vi "Facade.vi"(0 "Data In":T5, 2 "Display State In":T3, 3 "Container State":T4) -> (6 "Data Out":T5, 7 "Display State Out":T3, 8 "Action":T2)   [LabVIEW 2020, in "Termination XCtrl.xctl"]
uses:
  Termination XCtrl.xctl
  <vilib>/_xctls/Action.ctl
  <vilib>/_xctls/XControlSupport.lvlib
  Classes/Termination/Termination.lvclass
  <vilib>/_xctls/Container State.ctl
  Data.vi
  State.vi
panel:
  in  "Color Box":u32(colorbox)
  in  "Result":string
  in  "Tab":enum32{"End", "Finish", "TTL"}(tab)
  in  "Tmin":dbl caption="but wait at least (ms)" min=0.0 step=1.0
  in  "End on rep?":bool caption="end on rep boundary"
  in  "Tttl":string caption="min interval (ms)"
  in  "Nttl":i32 caption="max triggers" min=0 step=1
  in  "TermAction":T1(ring) caption="When true"
  in  "Latency":dbl caption="Response latency (ms)" min=0.0 step=1.0
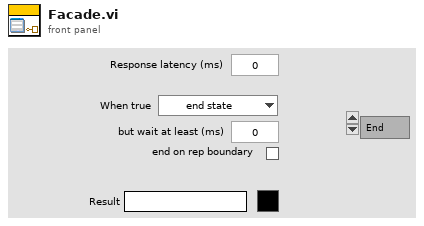
[diagram p1: front panel]
types:
  T1 = enum16{"end state", "let state finish", "TTL only"}
  T2 = typedef "XControlSupport.lvlib/Action.ctl" = cluster{"Data Changed?":bool, "State Changed?":bool, "Action Name":string}
  T3 = typedef "Termination XCtrl.xctl/State.vi" = cluster{"Numeric":dbl}
  T4 = typedef "XControlSupport.lvlib/Container State.ctl" = cluster{"Indicator?":bool, "Run Mode?":bool, " Refnum":refnum<vi>}
  T5 = typedef "Termination XCtrl.xctl/Data.vi" = refnum<class "Termination.lvclass">
  T6 = typedef "Tosca-Termination Condition Action.ctl" = enum16{"End state", "Complete state", "TTL only"}
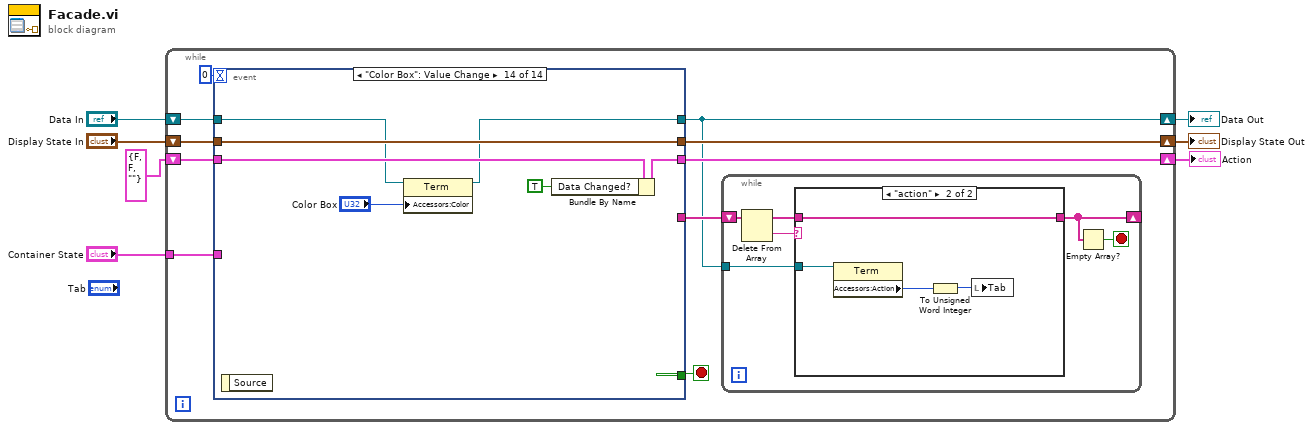
[diagram p0: block diagram]
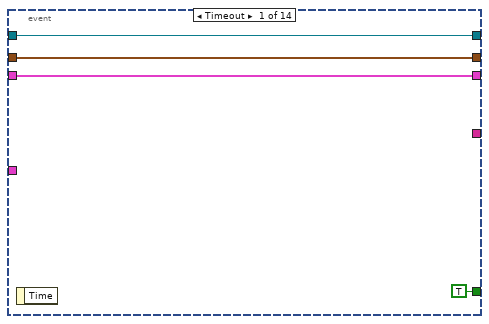
[diagram p3: hidden frame]
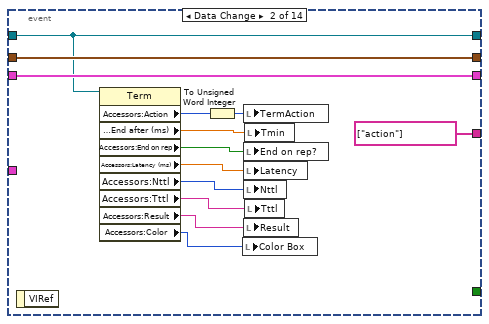
[diagram p4: hidden frame]
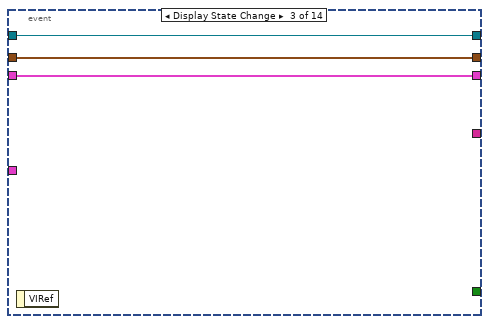
[diagram p5: hidden frame]
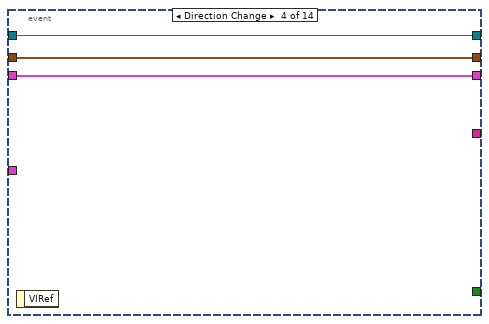
[diagram p6: hidden frame]
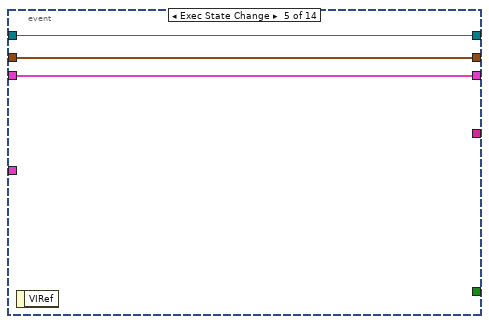
[diagram p7: hidden frame]
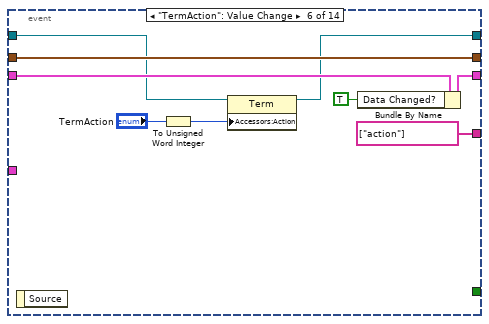
[diagram p8: hidden frame]
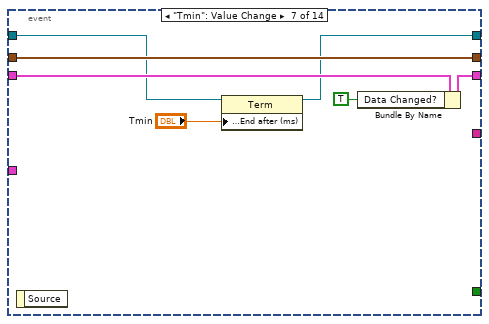
[diagram p9: hidden frame]
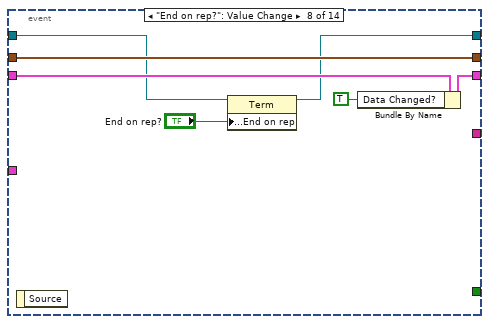
[diagram p10: hidden frame]
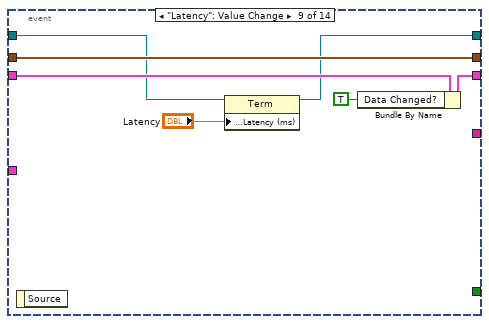
[diagram p11: hidden frame]
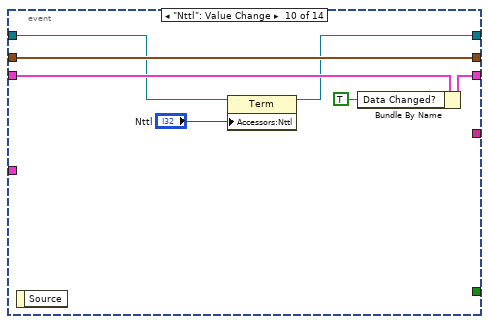
[diagram p12: hidden frame]
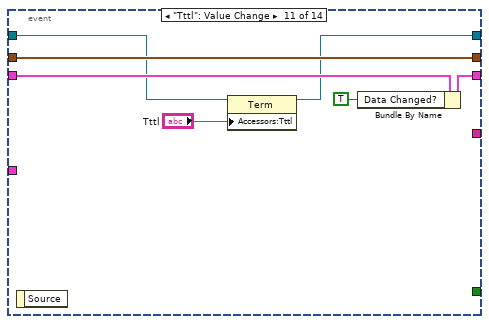
[diagram p13: hidden frame]
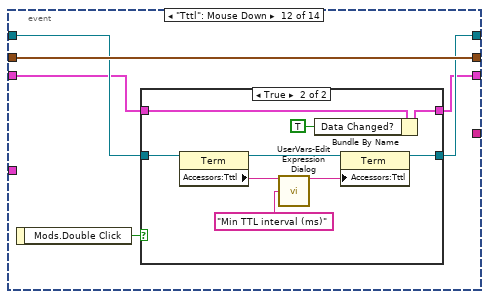
[diagram p14: hidden frame]
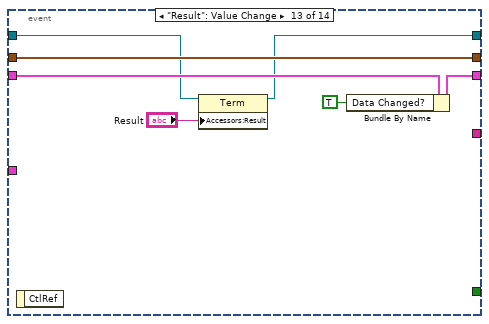
[diagram p16: hidden frame]
diagram:
  n1 = while {
    shift-right: [w16] -> w4
    shift-left: "Display State In" -> [w17]
    tunnel: "Container State" -> [w13]
    shift-right: [w8] -> w7
    shift-left: "Data In" -> [w12]
    shift-right: [w10] -> w2
    shift-left: T2 {"Data Changed?"=FALSE, "State Changed?"=FALSE, "Action Name"=""} ("Action") -> [w11]
    stop <- w15 stop-if-true
    n2 = event shown="[13] \"Color Box\": Value Change" {
      selector: _ -> [_ _ _ _ _ _ _ _ _ _ _ _ _ _]
      dyn-events: _ -> [_ _ _ _ _ _ _ _ _ _ _ _ _ _]
      timeout: 0 -> [_ _ _ _ _ _ _ _ _ _ _ _ _ _]
      tunnel: w17 -> [w31 w45 w48 w51 w54 w63 w70 w77 w84 w91 w98 w104 w122 w129]
      tunnel: [w31 w45 w48 w51 w54 w63 w70 w77 w84 w91 w98 w104 w122 w129] -> w16
      tunnel: [TRUE _ _ _ _ _ _ _ _ _ _ _ _ _] -> w15
      tunnel: w13 -> [_ _ _ _ _ _ _ _ _ _ _ _ _ _]
      tunnel: w12 -> [w29 w35 w47 w50 w53 w58 w66 w73 w80 w87 w94 w102 w119 w127]
      tunnel: [w29 w35 w47 w50 w53 w57 w65 w72 w79 w86 w93 w101 w118 w126] -> w8
      tunnel: [w30 w44 w46 w49 w52 w60 w68 w75 w82 w89 w96 w99 w117 w125] -> w10
      tunnel: w11 -> [w30 w44 w46 w49 w52 w62 w69 w76 w83 w90 w97 w100 w121 w128]
      tunnel: [_ string[] ["action"] _ _ _ string[] ["action"] _ _ _ _ _ _ _ _] -> w9
      event Timeout {
        n3 = event-data() -> ()  [unwired: 1 in, 1 out]
      }
      event Data Change {
        n4 = event-data() -> ()  [unwired: 1 in, 1 out]
        n5 = property class="Term"(reference=w35) -> ("Accessors:Action"=w42:T6, "Accessors:End after (ms)"=w39:dbl, "Accessors:End on rep"=w38:bool, "Accessors:Latency (ms)"=w37:dbl, "Accessors:Nttl"=w36:i32, "Accessors:Tttl"=w40:string, "Accessors:Result"=w34:string, "Accessors:Color"=w33:u32)  [unwired: 1 in, 2 out]
        n6 = To Unsigned Word Integer(number=w42) -> (unsigned 16bit integer=w41:u16)
        n7 = local write "Color Box"(w33) -> ()
        n8 = local write "TermAction"(w41) -> ()
        n9 = local write "End on rep?"(w38) -> ()
        n10 = local write "Latency"(w37) -> ()
        n11 = local write "Nttl"(w36) -> ()
        n12 = local write "Result"(w34) -> ()
        n13 = local write "Tmin"(w39) -> ()
        n14 = local write "Tttl"(w40) -> ()
      }
      event Display State Change {
        n15 = event-data() -> ()  [unwired: 1 in, 1 out]
      }
      event Direction Change {
        n16 = event-data() -> ()  [unwired: 1 in, 1 out]
      }
      event Exec State Change {
        n17 = event-data() -> ()  [unwired: 1 in, 1 out]
      }
      event "TermAction": Value Change {
        n18 = event-data() -> ()  [unwired: 1 in, 1 out]
        n19 = To Unsigned Word Integer(number="TermAction") -> (unsigned 16bit integer=w55:u16)
        n20 = property class="Term"(reference=w58, "Accessors:Action"=w55) -> (reference out=w57:T5)  [unwired: 1 in, 1 out]
        n21 = Bundle By Name(cluster=w62, "Data Changed?"=TRUE) -> (w60:T2)
      }
      event "Tmin": Value Change {
        n22 = event-data() -> ()  [unwired: 1 in, 1 out]
        n23 = property class="Term"(reference=w66, "Accessors:End after (ms)"="Tmin") -> (reference out=w65:T5)  [unwired: 1 in, 1 out]
        n24 = Bundle By Name(cluster=w69, "Data Changed?"=TRUE) -> (w68:T2)
      }
      event "End on rep?": Value Change {
        n25 = event-data() -> ()  [unwired: 1 in, 1 out]
        n26 = property class="Term"(reference=w73, "Accessors:End on rep"="End on rep?") -> (reference out=w72:T5)  [unwired: 1 in, 1 out]
        n27 = Bundle By Name(cluster=w76, "Data Changed?"=TRUE) -> (w75:T2)
      }
      event "Latency": Value Change {
        n28 = event-data() -> ()  [unwired: 1 in, 1 out]
        n29 = property class="Term"(reference=w80, "Accessors:Latency (ms)"="Latency") -> (reference out=w79:T5)  [unwired: 1 in, 1 out]
        n30 = Bundle By Name(cluster=w83, "Data Changed?"=TRUE) -> (w82:T2)
      }
      event "Nttl": Value Change {
        n31 = event-data() -> ()  [unwired: 1 in, 1 out]
        n32 = property class="Term"(reference=w87, "Accessors:Nttl"="Nttl") -> (reference out=w86:T5)  [unwired: 1 in, 1 out]
        n33 = Bundle By Name(cluster=w90, "Data Changed?"=TRUE) -> (w89:T2)
      }
      event "Tttl": Value Change {
        n34 = event-data() -> ()  [unwired: 1 in, 1 out]
        n35 = property class="Term"(reference=w94, "Accessors:Tttl"="Tttl") -> (reference out=w93:T5)  [unwired: 1 in, 1 out]
        n36 = Bundle By Name(cluster=w97, "Data Changed?"=TRUE) -> (w96:T2)
      }
      event "Tttl": Mouse Down {
        n37 = event-data() -> ("Mods.Double Click"=w103:bool)  [unwired: 1 in]
        n38 = case shown="True" w103 {
          tunnel: w102 -> [w106 w114]
          tunnel: [w106 w110] -> w101
          tunnel: w100 -> [w105 w109]
          tunnel: [w105 w108] -> w99
          frame False {
          }
          frame True {
            n39 = property class="Term"(reference=w114) -> (reference out=w112:T5, "Accessors:Tttl"=w113:string)  [unwired: 1 in, 1 out]
            n40 = call "UserVars-Edit Expression Dialog.vi"("Expr In"=w113, "Prompt"="Min TTL interval (ms)") -> ("Expr Out"=w111:string)  [unwired: 12 in, 1 out]
            n41 = Bundle By Name(cluster=w109, "Data Changed?"=TRUE) -> (w108:T2)
            n42 = property class="Term"(reference=w112, "Accessors:Tttl"=w111) -> (reference out=w110:T5)  [unwired: 1 in, 1 out]
          }
        }
      }
      event "Result": Value Change {
        n43 = event-data() -> ()  [unwired: 1 in, 1 out]
        n44 = property class="Term"(reference=w119, "Accessors:Result"="Result") -> (reference out=w118:T5)  [unwired: 1 in, 1 out]
        n45 = Bundle By Name(cluster=w121, "Data Changed?"=TRUE) -> (w117:T2)
      }
      event "Color Box": Value Change {
        n46 = event-data() -> ()  [unwired: 1 in, 1 out]
        n47 = property class="Term"(reference=w127, "Accessors:Color"="Color Box") -> (reference out=w126:T5)  [unwired: 1 in, 1 out]
        n48 = Bundle By Name(cluster=w128, "Data Changed?"=TRUE) -> (w125:T2)
      }
    }
    n49 = while {
      shift-right: [w20] -> _
      shift-left: w9 -> [w23]
      tunnel: w8 -> [w18]
      stop <- w19 stop-if-true
      n50 = Delete From Array(array=w23) -> (deleted portion=w21:string, array with subset deleted=w22:string[])  [unwired: 2 in]
      n51 = case shown="\"action\"" w21 {
        tunnel: w22 -> [w24 w28]
        tunnel: [w24 w28] -> w20
        tunnel: w18 -> [_ w27]
        frame "", Default {
        }
        frame "action" {
          n52 = property class="Term"(reference=w27) -> ("Accessors:Action"=w26:T6)  [unwired: 1 in, 2 out]
          n53 = To Unsigned Word Integer(number=w26) -> (unsigned 16bit integer=w25:u16)
          n54 = local write "Tab"(w25) -> ()
        }
      }
      n55 = Empty Array?(array=w20) -> (empty?=w19:bool)
    }
  }
  "Display State Out" <- w4
  "Data Out" <- w7
  "Action" <- w2
